vi "uActor_Exec.vi"(6 "Original uMsg":refnum<class "uMsg.lvclass">, 8 "error in (no error)":errorcluster, 9 "Data":refnum<class "uData.lvclass">, 10 "Command":string, 11 "Test_uActor_Echo in":refnum<class "Test_uActor_Echo.lvclass">) -> (0 "error out":errorcluster, 1 "reply":refnum<class "uData.lvclass">, 3 "Test_uActor_Echo out":refnum<class "Test_uActor_Echo.lvclass">)   [LabVIEW 2021, in "Test_uActor_Echo.lvclass"]
doc: "Dynamic dispatch method to allow children actors to handle incoming string commands.\n\nThe parent method returns an error if it receives an unknown incoming command."
uses:
  Test_uActor_Echo.lvclass
  Test_uActor_Echo.lvclass/Test_uActor_Echo.ctl
  Bin/uData.lvlibp/uData.lvclass
  Bin/uFramework.lvlibp/uMsg/uMsg.lvclass
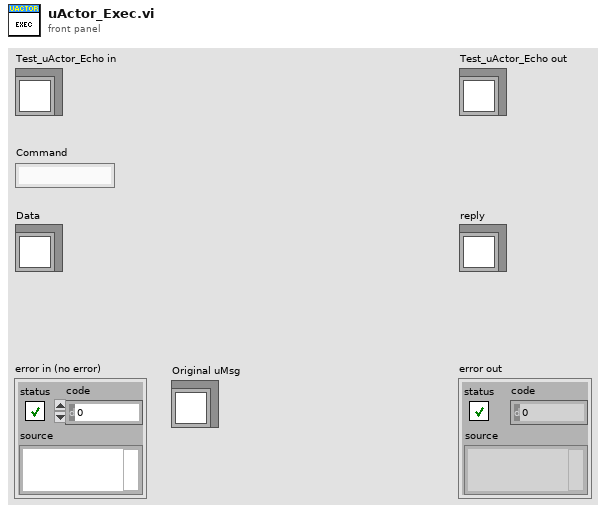
[diagram p1: front panel]
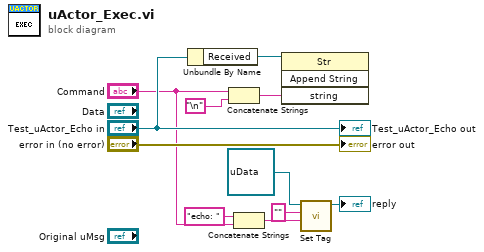
[diagram p0: block diagram]
diagram:
  n1 = Unbundle By Name("Test_uActor_Echo in") -> ("Received"=w11:refnum<vi>)
  n2 = Concatenate Strings("Command", "\n") -> (w8:string)
  n3 = Concatenate Strings("echo: " ("string"), "Command") -> (w2:string)
  n4 = invoke class="Str" method="Append String"(reference=w11, "string"=w8) -> ()  [unwired: 2 in, 4 out]
  n5 = call "Set Tag.vi"("Variant"=w2, "tag (case insensitive)"="", "uData in"=refnum<class "uData.lvclass"> refnum) -> ("uData out"=→"reply":refnum<class "uData.lvclass">)  [unwired: 6 in, 2 out]
  "error out" <- "error in (no error)"
  "Test_uActor_Echo out" <- "Test_uActor_Echo in"
